vi "arduino_serial_interface.vi"() -> ()   [LabVIEW 2018]
uses:
  <vilib>/Analysis/baseanly.llb/Mean (DBL).vi
  <vilib>/Instr/_visa.llb/VISA Configure Serial Port (Instr).vi
  <vilib>/Analysis/NI_AALBase.lvlib
panel:
  in  "Zero select":path
  out "Ave D":dbl
  out "Ave C":dbl
  out "Ave B":dbl
  out "Ave A":dbl
  out "Ave T":dbl
  out "Boolean 2":bool
  out "Boolean":bool
  in  "t3 (ms)":dbl
  in  "t2 (ms)":dbl
  in  "t1 (ms)":dbl
  out "appended array":dbl[](array[numeric])
  in  "milliseconds to wait":u32=10
  in  "Go MoE":dbl=0.05
  in  "Go Target":dbl=0.3
  in  "Steady Target":dbl=0.1
  in  "Auto Save":bool=TRUE
  out "Max T":dbl
  out "Time":dbl
  in  "MVC":dbl
  in  "Task":u16(ring) items=["[0] Callibration", "[1] MVC", "[2] Steady", "[3] Go", "[4] Randomized Inhibition"]
  out "File Name":string
  in  "Subject Number":i32
  out "Trial Number":i32
  in  "base path":path=path "C:/Users/cherukus/Desktop/TEST"
  in  "Save Button":bool
  out "T Array":dbl[](array[numeric])
  out "XY Graph":cluster{dbl[], dbl[]}[](graph)
  out "Plot Array":dbl[][](array[numeric])
  out "Read Array":dbl[][](array[numeric])
  out "Reading":bool
  out "Available?":bool
  out "Bytes in Buffer":u32
  out "Read Console":string
  in  "Process Stop Button":bool
  in  "TF":bool
  in  "TO":bool
  in  "COM Port":refnum<visa-resource-name>="COM5"
  in  "Baud Rate":u32=9600
  # "Arduino"
  # "USB Control"
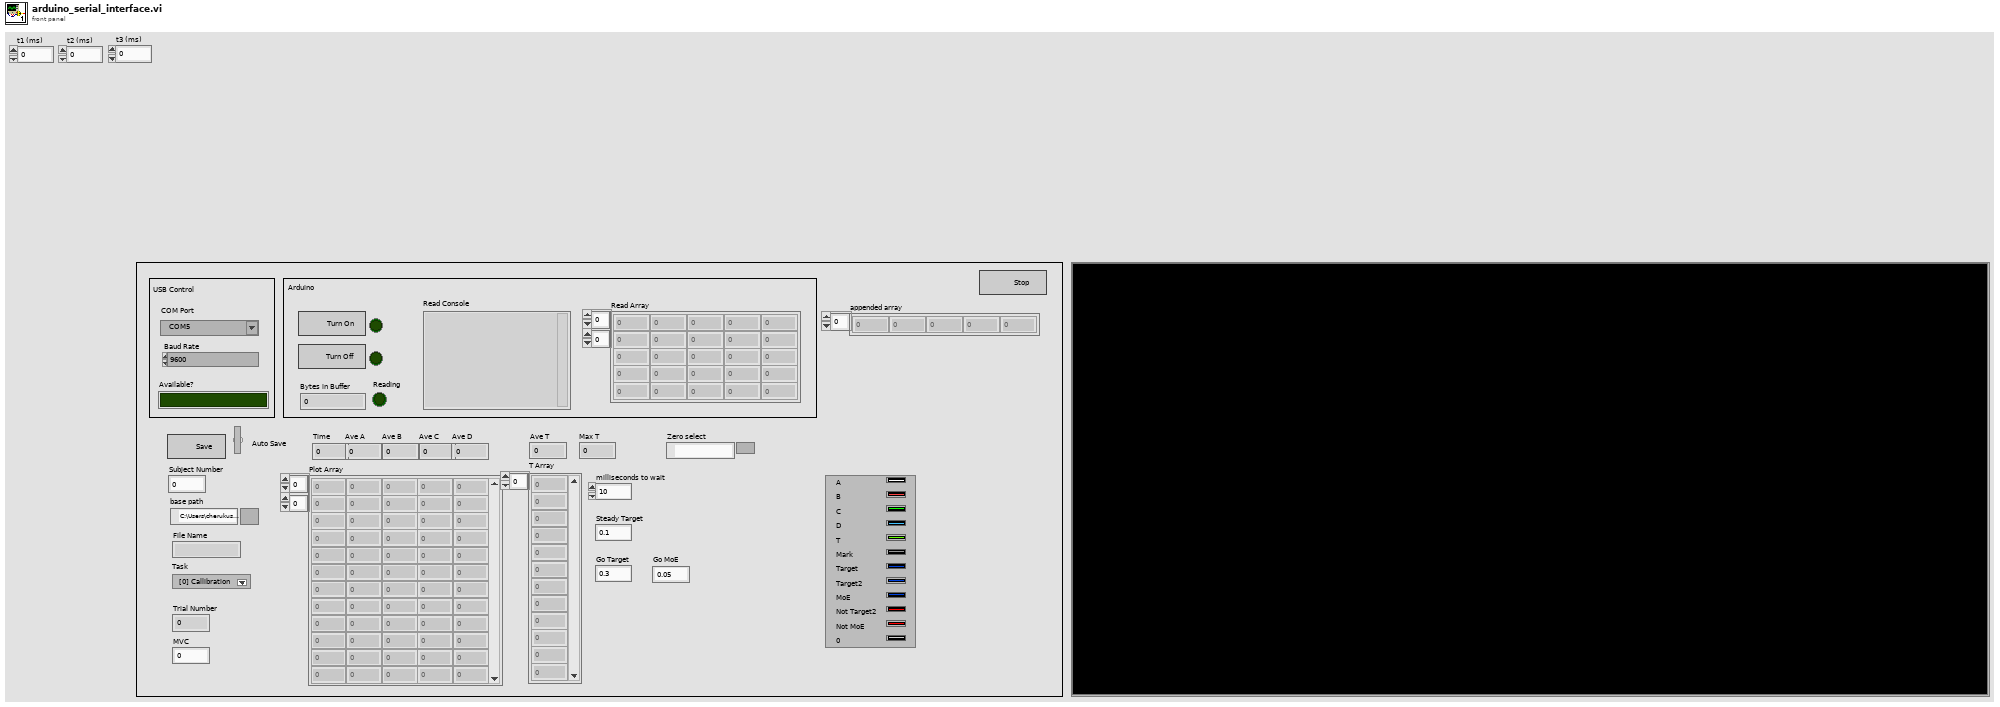
[diagram p1: front panel]
types:
  T1 = enum16{"open", "replace", "create", "open or create", "replace or create", "replace or create with confirmation"}
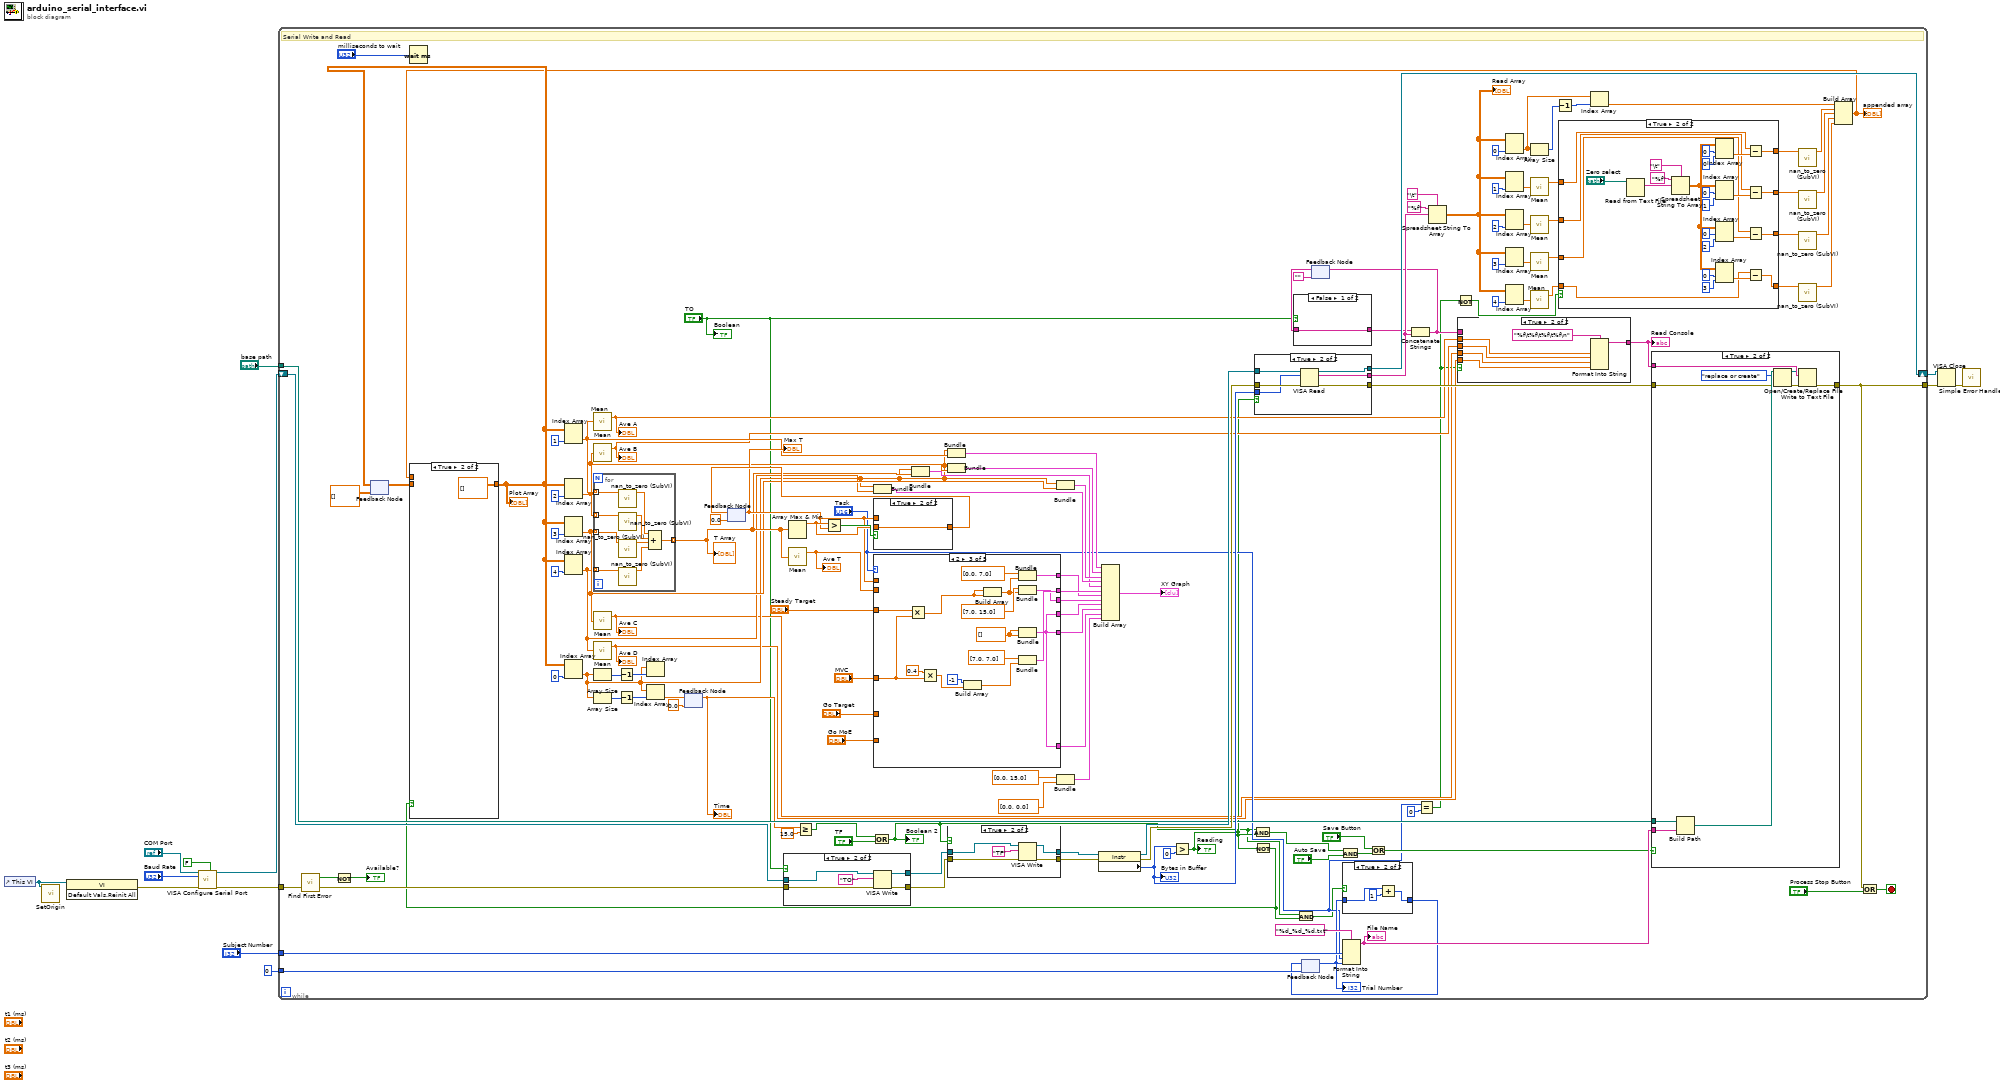
[diagram p0: block diagram]
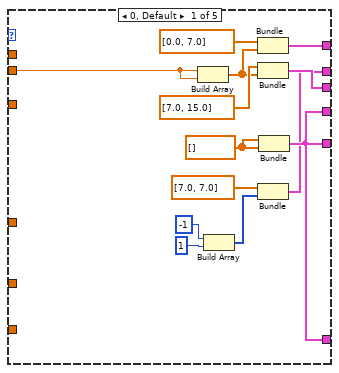
[diagram p4: hidden frame]
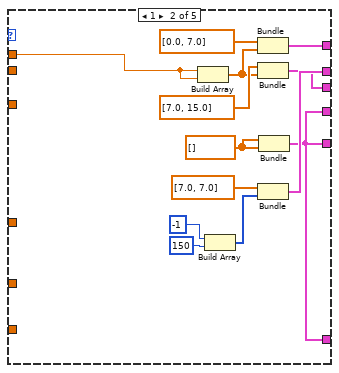
[diagram p5: hidden frame]
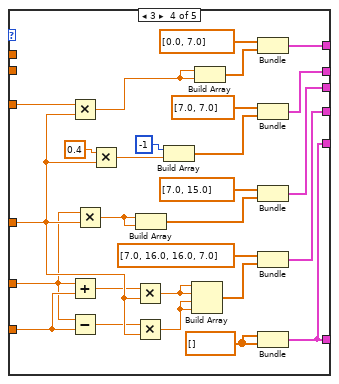
[diagram p6: hidden frame]
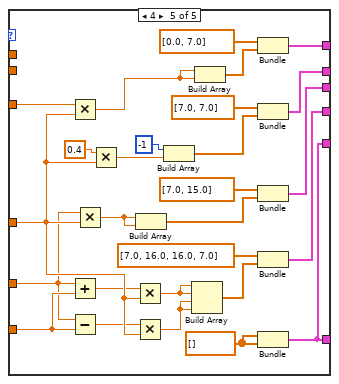
[diagram p7: hidden frame]
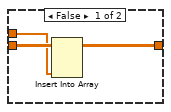
[diagram p9: hidden frame]
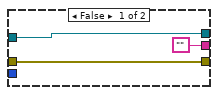
[diagram p11: hidden frame]
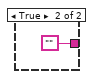
[diagram p13: hidden frame]
diagram:
  n1 = control-ref of="This VI"() -> (w2:refnum<vi>)
  n2 = call "SetOrigin.vi"("VI in"=w2) -> ()  [unwired: 10 in, 1 out]
  n3 = invoke class="VI" method="Default Vals.Reinit All"(reference=w2) -> (error out=w8:errorcluster)  [unwired: 2 in, 2 out]
  n4 = call-poly "VISA Configure Serial Port"("VISA resource name"="COM Port", "Enable Termination\nChar (T)"=FALSE ("Enable Termination\nChar (T)"), "baud rate (9600)"="Baud Rate", "error in (no error)"=w8) -> ("VISA resource name out"=w6:refnum<visa-resource-name>, "error out"=w7:errorcluster)  [unwired: 10 in]
  n5 = while {
    tunnel: [w132] -> w12
    tunnel: w7 -> [w136]
    shift-right: [w114] -> w13
    shift-left: w6 -> [w130]
    tunnel: "base path" -> [w113]
    tunnel: "Subject Number" -> [w109]
    tunnel: 0 -> [w95]
    stop <- w131 stop-if-true
    # "Serial Write and Read"
    n6 = call <vilib>:"Find First Error.vi"("error in (no error)"=w136) -> ("error out"=w135:errorcluster, "error?"=w134:bool)  [unwired: 3 in]
    n7 = Not(x=w134) -> (.not. x?=→"Available?":bool)
    n8 = feedback #1(dbl[][] [] ("array")) -> (w96:dbl[][])
    n9 = Wait (ms)(milliseconds to wait="milliseconds to wait") -> ()  [unwired: 1 out]
    n10 = feedback #2(0.0) -> (w99:dbl)
    "Time" <- w99
    n11 = feedback #3(0.0) -> (w78:dbl)
    "Max T" <- w78
    n12 = case shown="True" "TO" {
      tunnel: [w322 w327] -> w141
      tunnel: [w321 w326] -> w140
      tunnel: w130 -> [w322 w325]
      tunnel: w135 -> [w321 w323]
      frame False {
      }
      frame True {
        n13 = VISA Write(VISA resource name=w325, write buffer="TO", error in (no error)=w323) -> (VISA resource name out=w327:refnum<visa-resource-name>, error out=w326:errorcluster)  [unwired: 1 out]
      }
    }
    n14 = Greater Or Equal?(x=w99, y=15.0) -> (x >= y?=w100:bool)
    n15 = Or(x=w100, y="TF") -> (x .or. y?=w27:bool)
    "Boolean 2" <- w27
    n16 = case shown="True" w27 {
      tunnel: w141 -> [w314 w320]
      tunnel: w140 -> [w315 w317]
      tunnel: [w315 w316] -> w138
      tunnel: [w314 w319] -> w139
      frame False {
      }
      frame True {
        n17 = VISA Write(VISA resource name=w320, write buffer="TF", error in (no error)=w317) -> (VISA resource name out=w319:refnum<visa-resource-name>, error out=w316:errorcluster)  [unwired: 1 out]
      }
    }
    n18 = Bundle("array"=dbl[] [0.0, 15.0], "array"=dbl[] [0.0, 0.0]) -> (w75:cluster{"array":dbl[], "array":dbl[]})  [unwired: 1 in]
    n19 = property class="Instr"(reference=w139, error in=w138) -> (reference out=w117:refnum<visa-resource-name>, error out=w119:errorcluster, "Serial Settings:Number of Bytes at Serial Port"=w118:u32)
    "Bytes in Buffer" <- w118
    n20 = Greater?(x=w118, y=u32 0 ("x")) -> (0:w29:bool)
    "Reading" <- w29
    n21 = And(x=w27, y=w29) -> (x .and. y?=w31:bool)
    n22 = Not(x=w29) -> (.not. x?=w26:bool)
    n23 = case shown="True" w29 {
      tunnel: w119 -> [w285 w292]
      tunnel: w118 -> [_ w291]
      tunnel: w117 -> [w286 w290]
      tunnel: [w285 w289] -> w116
      tunnel: ["" w288] -> w115
      tunnel: [w286 w287] -> w114
      frame False {
      }
      frame True {
        n24 = VISA Read(VISA resource name=w290, byte count=w291, error in (no error)=w292) -> (VISA resource name out=w287:refnum<visa-resource-name>, read buffer=w288:string, error out=w289:errorcluster)  [unwired: 1 out]
      }
    }
    n25 = And(x=w27, y=w26) -> (x .and. y?=w28:bool)
    n26 = feedback #4(w95) -> (w94:i32)
    "Trial Number" <- w94
    n27 = feedback #5("") -> (w111:string)
    n28 = case shown="False" "TO" {
      tunnel: [w312 ""] -> w112
      tunnel: w111 -> [w312 _]
      frame False {
      }
      frame True {
      }
    }
    n29 = And(x=w31, y="Auto Save") -> (x .and. y?=w86:bool)
    n30 = case shown="True" w28 {
      tunnel: [w280 w283] -> w93
      tunnel: w94 -> [w280 w282]
      frame False {
      }
      frame True {
        n31 = Add(x=w282, y=1) -> (x+y=w283:i32)
      }
    }
    n32 = feedback-in #4(w93) -> ()
    n33 = Format Into String(format string="%d_%d_%d.txt", w109, "Task", w94) -> (resulting string=w108:string)  [unwired: 2 in, 1 out]
    "File Name" <- w108
    n34 = Or(x="Save Button", y=w86) -> (x .or. y?=w52:bool)
    n35 = Concatenate Strings(w112, w115) -> (w39:string)
    n36 = feedback-in #5(w39) -> ()
    n37 = Equal?(x="Task", y=u16 0) -> (x = y?=w24:bool)
    n38 = Spreadsheet String To Array(delimiter (Tab)="\t", format string="%f", spreadsheet string=w115) -> (array=w36:dbl[][])  [unwired: 1 in]
    "Read Array" <- w36
    n39 = Not(x=w24) -> (.not. x?=w23:bool)
    n40 = Index Array(array=w36, index (col)=0 ("disabled index (col)")) -> (element=w58:dbl[])  [unwired: 1 in]
    n41 = Index Array(array=w36, index (col)=1 ("disabled index (col)")) -> (element=w64:dbl[])  [unwired: 1 in]
    n42 = Index Array(array=w36, index (col)=2 ("disabled index (col)")) -> (element=w63:dbl[])  [unwired: 1 in]
    n43 = Index Array(array=w36, index (col)=3 ("disabled index (col)")) -> (element=w61:dbl[])  [unwired: 1 in]
    n44 = Index Array(array=w36, index (col)=4 ("disabled index (col)")) -> (element=w60:dbl[])  [unwired: 1 in]
    n45 = Array Size(array=w58) -> (size(s)=w59:i32)
    n46 = call-poly <vilib>:"Mean.vi"("X"=w64) -> ("mean"=w22:dbl)  [unwired: 1 out]
    n47 = call-poly <vilib>:"Mean.vi"("X"=w63) -> ("mean"=w19:dbl)  [unwired: 1 out]
    n48 = call-poly <vilib>:"Mean.vi"("X"=w61) -> ("mean"=w15:dbl)  [unwired: 1 out]
    n49 = call-poly <vilib>:"Mean.vi"("X"=w60) -> ("mean"=w14:dbl)  [unwired: 1 out]
    n50 = Decrement(x=w59) -> (x-1=w57:i32)
    n51 = case shown="True" w23 {
      tunnel: w22 -> [w145 w163]
      tunnel: [w145 w162] -> w21
      tunnel: w19 -> [w144 w158]
      tunnel: [w144 w157] -> w18
      tunnel: [w143 w156] -> w17
      tunnel: [w142 w155] -> w16
      tunnel: w15 -> [w143 w147]
      tunnel: w14 -> [w142 w146]
      frame False {
      }
      frame True {
        n52 = Read from Text File(file (use dialog)="Zero select") -> (text=w169:string)  [unwired: 3 in, 3 out]
        n53 = Spreadsheet String To Array(delimiter (Tab)="\t", format string="%f", spreadsheet string=w169) -> (array=w154:dbl[][])  [unwired: 1 in]
        n54 = Index Array(array=w154, index (row)=0 ("disabled index (row)"), index (col)=0 ("disabled index (col)")) -> (element=w164:dbl)
        n55 = Index Array(array=w154, index (row)=0, index (col)=1 ("disabled index (col)")) -> (element=w159:dbl)
        n56 = Index Array(array=w154, index (row)=0, index (col)=2 ("disabled index (col)")) -> (element=w149:dbl)
        n57 = Index Array(array=w154, index (row)=0, index (col)=3 ("disabled index (col)")) -> (element=w148:dbl)
        n58 = Subtract(x=w163, y=w164) -> (x-y=w162:dbl)
        n59 = Subtract(x=w158, y=w159) -> (x-y=w157:dbl)
        n60 = Subtract(x=w147, y=w149) -> (x-y=w156:dbl)
        n61 = Subtract(x=w146, y=w148) -> (x-y=w155:dbl)
      }
    }
    n62 = Index Array(array=w58, index=w57) -> (element=w51:dbl)
    n63 = call "nan_to_zero (SubVI).vi"("Numeric in"=w21) -> ("Numeric out"=w20:dbl)  [unwired: 10 in]
    n64 = call "nan_to_zero (SubVI).vi"("Numeric in"=w18) -> ("Numeric out"=w55:dbl)  [unwired: 10 in]
    n65 = call "nan_to_zero (SubVI).vi"("Numeric in"=w17) -> ("Numeric out"=w54:dbl)  [unwired: 10 in]
    n66 = call "nan_to_zero (SubVI).vi"("Numeric in"=w16) -> ("Numeric out"=w53:dbl)  [unwired: 10 in]
    n67 = Build Array(w51, w20, w55, w54, w53) -> (w56:dbl[])
    "appended array" <- w56
    n68 = case shown="True" w26 {
      tunnel: [w278 dbl[][] [] ("array")] -> w98
      tunnel: w96 -> [w277 _]
      tunnel: w56 -> [w276 _]
      frame False {
        n69 = Insert Into Array(array=w277, new element=w276) -> (w278:dbl[][])  [unwired: 2 in]
      }
      frame True {
      }
    }
    "Plot Array" <- w98
    n70 = feedback-in #1(w98) -> ()
    n71 = Index Array(array=w98, index (col)=1 ("disabled index (col)")) -> (element=w49:dbl[])  [unwired: 1 in]
    n72 = Index Array(array=w98, index (col)=2 ("disabled index (col)")) -> (element=w48:dbl[])  [unwired: 1 in]
    n73 = Index Array(array=w98, index (col)=3 ("disabled index (col)")) -> (element=w47:dbl[])  [unwired: 1 in]
    n74 = Index Array(array=w98, index (col)=4 ("disabled index (col)")) -> (element=w46:dbl[])  [unwired: 1 in]
    n75 = Index Array(array=w98, index (col)=0 ("disabled index (col)")) -> (element=w42:dbl[])  [unwired: 1 in]
    n76 = call-poly <vilib>:"Mean.vi"("X"=w49) -> ("mean"=w38:dbl)  [unwired: 1 out]
    "Ave A" <- w38
    n77 = call-poly <vilib>:"Mean.vi"("X"=w48) -> ("mean"=w35:dbl)  [unwired: 1 out]
    "Ave B" <- w35
    n78 = for {
      tunnel: [w311] -> w50 mode=indexing
      tunnel: w49 -> [w309] mode=indexing
      tunnel: w48 -> [w308] mode=indexing
      tunnel: w47 -> [w306] mode=indexing
      tunnel: w46 -> [w304] mode=indexing
      n79 = call "nan_to_zero (SubVI).vi"("Numeric in"=w309) -> ("Numeric out"=w310:dbl)  [unwired: 10 in]
      n80 = call "nan_to_zero (SubVI).vi"("Numeric in"=w308) -> ("Numeric out"=w307:dbl)  [unwired: 10 in]
      n81 = call "nan_to_zero (SubVI).vi"("Numeric in"=w306) -> ("Numeric out"=w305:dbl)  [unwired: 10 in]
      n82 = call "nan_to_zero (SubVI).vi"("Numeric in"=w304) -> ("Numeric out"=w303:dbl)  [unwired: 10 in]
      n83 = Compound Arithmetic op=ADD(w310, w307, w305, w303) -> (w311:dbl)
    }
    "T Array" <- w50
    n84 = call-poly <vilib>:"Mean.vi"("X"=w47) -> ("mean"=w34:dbl)  [unwired: 1 out]
    "Ave C" <- w34
    n85 = call-poly <vilib>:"Mean.vi"("X"=w46) -> ("mean"=w37:dbl)  [unwired: 1 out]
    "Ave D" <- w37
    n86 = Array Size(array=w42) -> (size(s)=w102:i32)
    n87 = Array Size(array=w42) -> (size(s)=w45:i32)
    n88 = Decrement(x=w102) -> (x-1=w103:i32)
    n89 = Decrement(x=w45) -> (x-1=w44:i32)
    n90 = Index Array(array=w42, index=w103) -> ()  [unwired: 1 out]
    n91 = Index Array(array=w42, index=w44) -> (element=w43:dbl)
    n92 = feedback-in #2(w43) -> ()
    n93 = Array Max & Min(array=w50) -> (max value=w82:dbl)  [unwired: 3 out]
    n94 = call-poly <vilib>:"Mean.vi"("X"=w50) -> ("mean"=w25:dbl)  [unwired: 1 out]
    "Ave T" <- w25
    n95 = Greater?(x=w82, y=w78) -> (0:w85:bool)
    n96 = Bundle("array"=w42, "array"=w46) -> (w121:cluster{"array":dbl[], "array":dbl[]})  [unwired: 1 in]
    n97 = case shown="True" w85 {
      tunnel: [w274 w275] -> w84
      tunnel: w82 -> [_ w275]
      tunnel: w78 -> [w274 _]
      frame False {
      }
      frame True {
      }
    }
    n98 = feedback-in #3(w84) -> ()
    n99 = case shown="2" "Task" {
      tunnel: [w179 w202 w218 w245 w272] -> w106
      tunnel: [w178 w201 w217 w244 w271] -> w105
      tunnel: [w181 w192 w205 w234 w261] -> w81
      tunnel: [w182 w196 w209 w231 w258] -> w80
      tunnel: "MVC" -> [_ _ w207 w225 w252]
      tunnel: w78 -> [_ w193 _ _ _]
      tunnel: [w181 w192 w205 w228 w255] -> w77
      tunnel: [w181 w192 w205 w228 w255] -> w76
      tunnel: "Steady Target" -> [_ _ w204 w221 w248]
      tunnel: "Go Target" -> [_ _ _ w220 w247]
      tunnel: "Go MoE" -> [_ _ _ w222 w249]
      tunnel: w25 -> [w183 _ _ _ _]
      frame 0, Default {
        w184 = dbl[] [] ("array")
        n100 = Build Array(w183, w183) -> (w185:dbl[])
        n101 = Build Array(-1, 1) -> (w187:i32[])
        n102 = Bundle("array"=dbl[] [0.0, 7.0], w185) -> (w178:cluster{"array":dbl[], dbl[]})  [unwired: 1 in]
        n103 = Bundle("array"=dbl[] [7.0, 15.0], w185) -> (w182:cluster{"array":dbl[], dbl[]})  [unwired: 1 in]
        n104 = Bundle("array"=dbl[] [7.0, 7.0], w187) -> (w179:cluster{"array":dbl[], i32[]})  [unwired: 1 in]
        n105 = Bundle("array"=w184, "array"=w184) -> (w181:cluster{"array":dbl[], "array":dbl[]})  [unwired: 1 in]
      }
      frame 1 {
        w194 = dbl[] [] ("array")
        n106 = Build Array(w193, w193) -> (w195:dbl[])
        n107 = Build Array(-1, 150) -> (w198:i32[])
        n108 = Bundle("array"=dbl[] [0.0, 7.0], w195) -> (w201:cluster{"array":dbl[], dbl[]})  [unwired: 1 in]
        n109 = Bundle("array"=dbl[] [7.0, 15.0], w195) -> (w196:cluster{"array":dbl[], dbl[]})  [unwired: 1 in]
        n110 = Bundle("array"=dbl[] [7.0, 7.0], w198) -> (w202:cluster{"array":dbl[], i32[]})  [unwired: 1 in]
        n111 = Bundle("array"=w194, "array"=w194) -> (w192:cluster{"array":dbl[], "array":dbl[]})  [unwired: 1 in]
      }
      frame 2 {
        w206 = dbl[] [] ("array")
        n112 = Multiply(x=w204, y=w207) -> (x*y=w210:dbl)
        n113 = Multiply(x=0.4, y=w207) -> (x*y=w213:dbl)
        n114 = Build Array(-1, w213) -> (w214:dbl[])
        n115 = Build Array(w210, w210) -> (w208:dbl[])
        n116 = Bundle("array"=dbl[] [0.0, 7.0], w208) -> (w217:cluster{"array":dbl[], dbl[]})  [unwired: 1 in]
        n117 = Bundle("array"=dbl[] [7.0, 15.0], w208) -> (w209:cluster{"array":dbl[], dbl[]})  [unwired: 1 in]
        n118 = Bundle("array"=dbl[] [7.0, 7.0], w214) -> (w218:cluster{"array":dbl[], dbl[]})  [unwired: 1 in]
        n119 = Bundle("array"=w206, "array"=w206) -> (w205:cluster{"array":dbl[], "array":dbl[]})  [unwired: 1 in]
      }
      frame 3 {
        w229 = dbl[] [] ("array")
        n120 = Multiply(x=w221, y=w225) -> (x*y=w232:dbl)
        n121 = Add(x=w220, y=w222) -> (x+y=w224:dbl)
        n122 = Subtract(x=w220, y=w222) -> (x-y=w223:dbl)
        n123 = Multiply(x=w220, y=w225) -> (x*y=w227:dbl)
        n124 = Multiply(x=0.4, y=w225) -> (x*y=w240:dbl)
        n125 = Multiply(x=w224, y=w225) -> (x*y=w235:dbl)
        n126 = Multiply(x=w223, y=w225) -> (x*y=w236:dbl)
        n127 = Build Array(w227, w227) -> (w226:dbl[])
        n128 = Build Array(-1, w240) -> (w241:dbl[])
        n129 = Build Array(w235, w235, w236, w236) -> (w237:dbl[])
        n130 = Build Array(w232, w232) -> (w230:dbl[])
        n131 = Bundle("array"=dbl[] [0.0, 7.0], w230) -> (w244:cluster{"array":dbl[], dbl[]})  [unwired: 1 in]
        n132 = Bundle("array"=dbl[] [7.0, 7.0], w241) -> (w245:cluster{"array":dbl[], dbl[]})  [unwired: 1 in]
        n133 = Bundle("array"=dbl[] [7.0, 15.0], w226) -> (w231:cluster{"array":dbl[], dbl[]})  [unwired: 1 in]
        n134 = Bundle("array"=dbl[] [7.0, 16.0, 16.0, 7.0], w237) -> (w234:cluster{"array":dbl[], dbl[]})  [unwired: 1 in]
        n135 = Bundle("array"=w229, "array"=w229) -> (w228:cluster{"array":dbl[], "array":dbl[]})  [unwired: 1 in]
      }
      frame 4 {
        w256 = dbl[] [] ("array")
        n136 = Multiply(x=w248, y=w252) -> (x*y=w259:dbl)
        n137 = Add(x=w247, y=w249) -> (x+y=w251:dbl)
        n138 = Subtract(x=w247, y=w249) -> (x-y=w250:dbl)
        n139 = Multiply(x=w247, y=w252) -> (x*y=w254:dbl)
        n140 = Multiply(x=0.4, y=w252) -> (x*y=w267:dbl)
        n141 = Multiply(x=w251, y=w252) -> (x*y=w262:dbl)
        n142 = Multiply(x=w250, y=w252) -> (x*y=w263:dbl)
        n143 = Build Array(w254, w254) -> (w253:dbl[])
        n144 = Build Array(-1, w267) -> (w268:dbl[])
        n145 = Build Array(w262, w262, w263, w263) -> (w264:dbl[])
        n146 = Build Array(w259, w259) -> (w257:dbl[])
        n147 = Bundle("array"=dbl[] [0.0, 7.0], w257) -> (w271:cluster{"array":dbl[], dbl[]})  [unwired: 1 in]
        n148 = Bundle("array"=dbl[] [7.0, 7.0], w268) -> (w272:cluster{"array":dbl[], dbl[]})  [unwired: 1 in]
        n149 = Bundle("array"=dbl[] [7.0, 15.0], w253) -> (w258:cluster{"array":dbl[], dbl[]})  [unwired: 1 in]
        n150 = Bundle("array"=dbl[] [7.0, 16.0, 16.0, 7.0], w264) -> (w261:cluster{"array":dbl[], dbl[]})  [unwired: 1 in]
        n151 = Bundle("array"=w256, "array"=w256) -> (w255:cluster{"array":dbl[], "array":dbl[]})  [unwired: 1 in]
      }
    }
    n152 = Bundle("array"=w42, w50) -> (w120:cluster{"array":dbl[], dbl[]})  [unwired: 1 in]
    n153 = Bundle("array"=w42, "array"=w49) -> (w124:cluster{"array":dbl[], "array":dbl[]})  [unwired: 1 in]
    n154 = Bundle("array"=w42, "array"=w48) -> (w123:cluster{"array":dbl[], "array":dbl[]})  [unwired: 1 in]
    n155 = Bundle("array"=w42, "array"=w47) -> (w122:cluster{"array":dbl[], "array":dbl[]})  [unwired: 1 in]
    n156 = Build Array(w124, w123, w122, w121, w120, w106, w105, w80, w81, w77, w76, w75) -> (→"XY Graph":cluster{"array":dbl[], "array":dbl[]}[])
    n157 = case shown="True" w24 {
      tunnel: [w171 w172] -> w30
      tunnel: w39 -> [w171 _]
      tunnel: w38 -> [_ w176]
      tunnel: w37 -> [_ w175]
      tunnel: w35 -> [_ w174]
      tunnel: w34 -> [_ w173]
      frame False {
      }
      frame True {
        n158 = Format Into String(format string="%f\t%f\t%f\t%f\n", w176, w174, w173, w175) -> (resulting string=w172:string)  [unwired: 2 in, 1 out]
      }
    }
    "Read Console" <- w30
    n159 = case shown="True" w52 {
      tunnel: w30 -> [_ w302]
      tunnel: w116 -> [w293 w299]
      tunnel: [w293 w301] -> w132
      tunnel: w113 -> [_ w296]
      tunnel: w108 -> [_ w295]
      frame False {
      }
      frame True {
        n160 = Build Path(base path=w296, name or relative path=w295) -> (appended path=w300:path)
        n161 = Open/Create/Replace File(file path (use dialog)=w300, error in=w299, operation (0:open)=T1."replace or create") -> (refnum out=w297:refnum<file>, error out=w298:errorcluster)  [unwired: 3 in, 1 out]
        n162 = Write to Text File(file (use dialog)=w297, text=w302, error in=w298) -> (error out=w301:errorcluster)  [unwired: 1 in, 2 out]
      }
    }
    n163 = Or(x=w132, y="Process Stop Button") -> (x .or. y?=w131:bool)
    "Boolean" <- "TO"
  }
  n164 = VISA Close(VISA resource name=w13, error in (no error)=w12) -> (error out=w11:errorcluster)
  n165 = call <vilib>:"Simple Error Handler.vi"("error in (no error)"=w11) -> ()  [unwired: 4 in, 5 out]
